vi "PWM Out, Latched (subVI).vi"(0 "Low Period":u16=500, 2 "High Period":u16=500, 3 "Load":bool, 5 "Run":bool=TRUE) -> (7 "PWM Output":bool)   [LabVIEW 2015]
doc: "This subVI supports a latched PWM output. The Low Period and High Period controls (in ms) will be translated to a PWM output one period after the Load boolean is asserted. The Run boolean acts as a gate to output the generated pulse train to the PWM Output indicator."
panel:
  # "This subVI supports a latched PWM output.  The Low Period and High Period controls (in ms) will be translated to a PWM output one period after the Load boolean is asserted.  The Run boolean acts as a gate to output the generated pulse train to the PWM Output indicator."
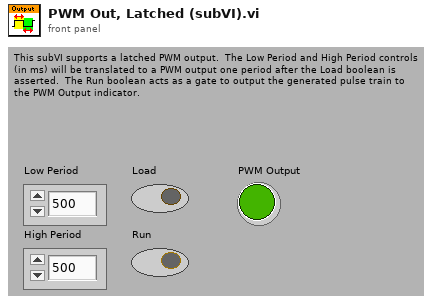
[diagram p1: front panel]
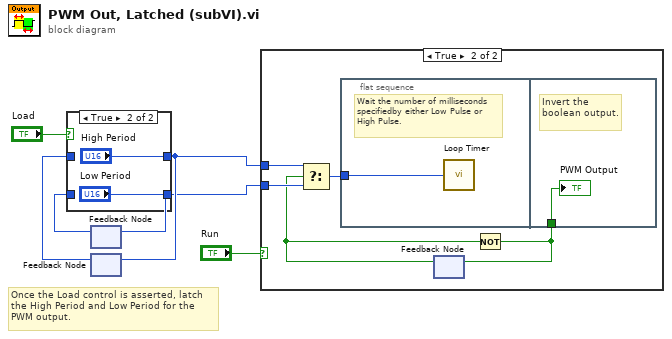
[diagram p0: block diagram]
diagram:
  # "Once the Load control is asserted, latch the High Period and Low Period for the PWM output."
  n1 = feedback #1() -> (w2:u16)  [unwired: 1 out]
  n2 = feedback #2() -> (w1:u16)  [unwired: 1 out]
  n3 = case shown="False" "Load" {
    tunnel: [w8 "High Period"] -> w4
    tunnel: [w7 "Low Period"] -> w3
    tunnel: w1 -> [w8 _]
    tunnel: w2 -> [w7 _]
    frame False {
    }
    frame True {
    }
  }
  n4 = feedback-in #1(w3) -> ()
  n5 = feedback-in #2(w4) -> ()
  n6 = case shown="False" "Run" {
    tunnel: w4 -> [_ w15]
    tunnel: w3 -> [_ w14]
    frame False {
    }
    frame True {
      n7 = flat-sequence {
        tunnel: w13 -> [w16]
        tunnel: w12 -> [w17]
        frame #0 {
          # "Wait the number of milliseconds specifiedby either Low Pulse or High Pulse."
          n8 = call "Loop Timer"("Count(mSec)"=w16) -> ()  [unwired: 1 out]
        }
        frame #1 {
          # "Invert the boolean output."
          "PWM Output" <- w17
        }
      }
      n9 = feedback #3() -> (w11:bool)  [unwired: 1 out]
      n10 = Select(t=w15, s=w11, f=w14) -> (s? t:f=w13:u16)
      n11 = Not(x=w11) -> (.not. x?=w12:bool)
      n12 = feedback-in #3(w12) -> ()
    }
  }
